vi "GetGXMLCfgCurrent.vi"(8 "error in (no error)":errorcluster, 11 "Current in":refnum<class "Current.lvclass">) -> (0 "error out":errorcluster, 2 "CurrentChanCfg":T1, 3 "Current out":refnum<class "Current.lvclass">)   [LabVIEW 2018, in "Measurement Channels.lvlib" / "Current.lvclass"]
uses:
  Current.lvclass
  CurrentProps_TD.ctl
  Current.lvclass/Current.ctl
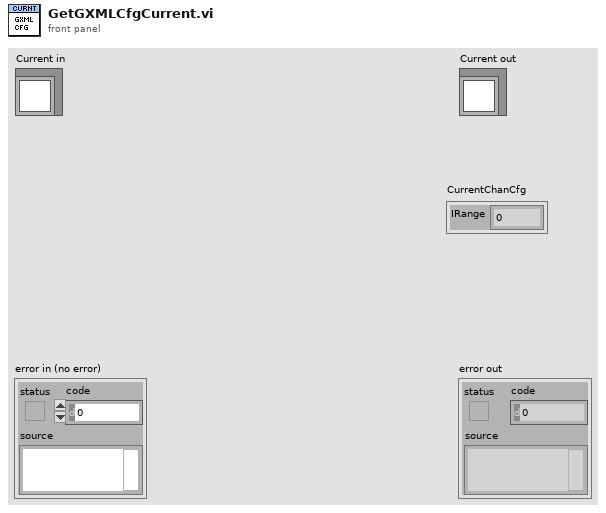
[diagram p1: front panel]
types:
  T1 = typedef "CurrentProps_TD.ctl" = cluster{"IRange":dbl}
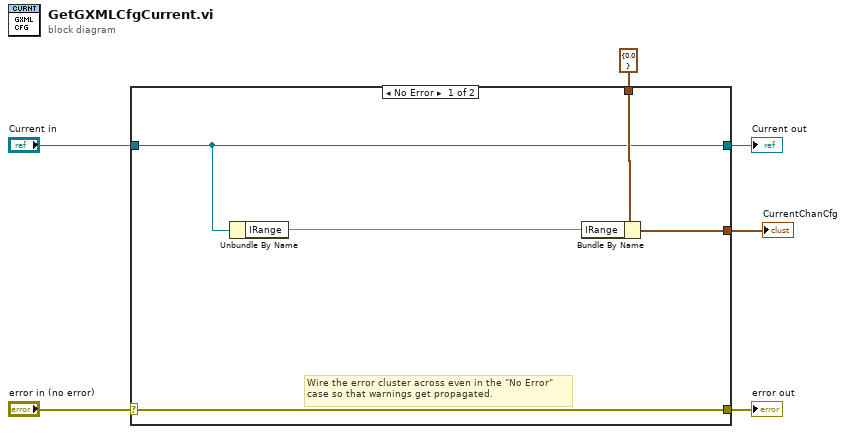
[diagram p0: block diagram]
diagram:
  n1 = case shown="No Error" "error in (no error)" {
    selector: "error in (no error)" -> [w11 w14]
    tunnel: [w11 w14] -> w5
    tunnel: [w8 w13] -> w3
    tunnel: "Current in" -> [w8 w13]
    tunnel: [w9 w12] -> w2
    tunnel: T1 {"IRange"=0.0} ("CurrentChanCfg") -> [w10 w12]
    frame No Error {
      # "Wire the error cluster across even in the \"No Error\"\ncase so that warnings get propagated."
      n2 = Unbundle By Name(w8) -> ("IRange"=w7:dbl)
      n3 = Bundle By Name(cluster=w10, "IRange"=w7) -> (w9:T1)
    }
    frame Error {
    }
  }
  "error out" <- w5
  "Current out" <- w3
  "CurrentChanCfg" <- w2
